vi "Synthetic_Jet_Optimisation.vi"() -> (5 "Plug in titles":string[](array[string]), 7 "Plug in values":string[](array[string]))   [LabVIEW 2011]
uses:
  Controls/SJ_Channels.ctl
  Controls/SJ_Data_Cluster.ctl
  <vilib>/Analysis/2dsp.llb/Integral Method.ctl
  Globals/Meas_global.vi
  Globals/Plug_in_data_global.vi
  <vilib>/Analysis/1siggen.llb/Ramp Pattern by Delta.vi
  <vilib>/Analysis/baseanly.llb/Scale 1D.vi
  <vilib>/Analysis/5stat.llb/RMS (DBL).vi
  <vilib>/Analysis/8numeric.llb/1D Numeric Integration.vi
  <vilib>/Analysis/baseanly.llb/Quick Scale 1D.vi
  <vilib>/Analysis/1siggen.llb/Ramp Pattern by Samples.vi
  Acquisition/Data_Translation/DataTranslation_global.vi
  <vilib>/Analysis/NI_AALBase.lvlib
  <vilib>/Analysis/NI_AALPro.lvlib
panel:
  out "subarray":dbl[][](array[numeric])
  out "output array 2":dbl[][][](array[numeric])
  out "output array":dbl[][][](array[numeric])
  out "Updated Amps":dbl[](array[numeric])
  out "Max Amp":dbl
  out "Min Amp":dbl
  out "Sweep Frequency":dbl[](array[numeric])
  out "Last Block in Genertation":bool
  out "Max Input Voltage _V_":dbl
  out "Blocks per Generation":i32
  out "Sweep Size":i32
  out "Number of Particles":i32
  out "ID Number":i32
  out "Number of Generations":i32
  out "Optimisation Type":i32
  out "Target Value":dbl
  out "Phase Average?":bool
  out "Samps per cyle":i32
  out "Formation Criteria":dbl
  out "Jet Formation":bool
  out "Strouhal Number":dbl
  out "Stokes Number":dbl
  out "nu":dbl=1.55e-05
  out "Omega":dbl=1200.0
  out "Reynolds Number":dbl
  out "Charicteristic Velocity m_s":dbl
  out "Stroke Length _m_":dbl
  out "Cavity:Helmholtz:Hz":dbl=428.16291209383184
  out "LEM Velocity _ms_":dbl[](array[numeric])=[3.7049856348371377, 3.4607988115264297, 3.0653584733968287, 2.5359472607578692, 1.895702983998723, 1.1726073902466658, 0.3982632267462864, -0.3934869508418966, -1.1680398605184126, -1.8915438234131698, -2.5323782445904723, -3.062535584780142, -3.458845424238726, -3.7039871212762807, -3.787246807411894, -3.7049856348371377, -3.4607988115264297, -3.0653584733968295, -2.5359472607578692, -1.8957029839987247, -1.172607390246666, -0.3982632267462887, 0.3934869508418962, 1.1680398605184101, 1.8915438234131694, 2.53237824459047, 3.0625355847801417, 3.4588454242387248, 3.7039871212762803, 3.7872468074118935]
  out "LEM Max Velocity _ms_":dbl=3.7872475686779676
  out "LEM Phase Velocity _deg_":dbl=-258.0363282123533
  out "Phase Pressure _deg_":dbl=-169.14507601114087
  out "Phase Velocity _deg_":dbl=373.1272896341652
  out "Phase Input Voltage _deg_":dbl=8.606071626556414
  out "Phase Angle _deg_":dbl[](array[numeric])=[0.0, 12.0, 24.0, 36.0, 48.0, 60.0, 72.0, 84.0, 96.0, 108.0, 120.0, 132.0, 144.0, 156.0, 168.0, 180.0, 192.0, 204.0, 216.0, 228.0, 240.0, 252.0, 264.0, 276.0, 288.0, 300.0, 312.0, 324.0, 336.0, 348.0]
  out "Amplitude (V)":dbl=70.0
  out "Frequency (Hz)":dbl=1200.0
  out "AS Freq":dbl=36036.04
  out "Output Data Names":string[](array[string])=["Max Pressure _Pa_", "Max Velocity m_s", "Max Current _A_", "Max Displacement _m_", "Phase Displ _deg_", "Phase Pressure _deg_", "Phase Velocity _deg_", "Phase Current _deg_", "Phase Input Voltage _deg_", "LEM Max Velocity _ms_", "LEM Phase Velocity _deg_"]
  out "Input Voltage _V_":dbl[](array[numeric])=[-5.5088632433799996, -12.651031578584, -19.235618350895997, -24.9961110527, -29.670494279084004, -33.04444558276, -35.005182361704, -35.409211536216006, -34.310616683552006, -31.700640287920002, -27.711473499856005, -22.510574222680006, -16.349366000988, -9.495663135284, -2.196569584672, 5.184714435096, 12.336113665324001, 18.917564300223997, 24.689891482827996, 29.395636083331993, 32.795741589576, 34.758786092276, 35.215182844328, 34.127830748423996, 31.539748142271996, 27.582652797175996, 22.404475723135995, 16.265220463328, 9.402109185388, 2.133489422836]
  out "Pressure _Pa_":dbl[](array[numeric])=[-27.3956675953706, 95.65286233449294, 217.28142105099454, 325.3916285730047, 412.49320713856633, 477.62511872885386, 518.8812420389512, 544.5955786383588, 546.2858417945154, 525.7943338813993, 485.98446016799124, 431.53940396868336, 357.29264741860004, 257.81676584697294, 146.44897730607346, 25.39291194062997, -95.29994862668336, -216.63005998968256, -325.4638615668826, -412.65459893301875, -477.423305725176, -519.6780076017092, -543.7330519967387, -544.6659346048561, -524.568602441649, -487.2326508157636, -435.0203186855821, -361.9795522274816, -267.2741357434412, -152.01151538796677]
  out "Zeros":dbl[](array[numeric])=[1.4978743085562871, 0.2341330189017041, -0.35175473981443495, 0.0022887999999999997, -3.0068544366899315, 2.8293]
  out "Velocity m_s":dbl[](array[numeric])=[-0.006589971422005106, -0.006419643065741468, -0.009111611844261746, -0.006030326884042168, -0.004272653157727323, -0.0068849933436421745, -0.010636233235274354, -0.0035467148583991693, -0.008496862890472292, -0.005357351691532665, -0.007065956289182962, -0.006648911559621155, -0.005058171342073957, -0.008830133605031026, -0.0038751674420970687, -0.005274584307176274, 0.000979796600094568, -0.005616008146962059, -0.00729733372181674, 0.0005036149760482819, -0.004633370846616606, -0.007598533001820504, -0.005354959759266961, -0.003855515705978843, -0.005082756078867318, -0.0008163141834672163, -0.007346968606858383, -0.00413574997102441, -0.00277648312445221, -0.00052352239052674]
  out "RMS Velocity m_s":dbl=0.014914535983039488 format="%0.2f"
  out "RMS Pressure _Pa_":dbl=395.7699897259115 format="%0.2f"
  out "Max Pressure _Pa_":dbl=546.2858417945154 format="%0.2f"
  out "Max Velocity m_s":dbl=0.000979796600094568
  in  "Menu Ring":u16(ring) items=["Max Pressure _Pa_", "", "Max Velocity m_s"]
  out "Frequency Plot":cluster{"Sweep Frequency":dbl[], dbl[]}[](graph)
  out "Pressure Plot":cluster{dbl[], dbl[]}[](graph)=[{[0.0, 12.0, 24.0, 36.0, 48.0, 60.0, 72.0, 84.0, 96.0, 108.0, 120.0, 132.0, 144.0, 156.0, 168.0, 180.0, 192.0, 204.0, 216.0, 228.0, 240.0, 252.0, 264.0, 276.0, 288.0, 300.0, 312.0, 324.0, 336.0, 348.0], [-0.15557712257291065, -0.35728080433659803, -0.5432376920119246, -0.705921142218441, -0.8379315153272326, -0.9332160799164545, -0.9885897155857659, -1.0, -0.9689743203815658, -0.8952653536353687, -0.7826063416157439, -0.6357265029653804, -0.4617263500562873, -0.2681692905127802, -0.06203384626131485, 0.1464227586596542, 0.34838713233438734, 0.5342554516040381, 0.697273122209331, 0.8301691793748806, 0.926192371045399, 0.9816311796924717, 0.9945203893712923, 0.9638122191316959, 0.8907215601232357, 0.7789682853842954, 0.632730149899583, 0.45934997583022086, 0.26552721106968635, 0.060252384345070756]}, {[0.0, 12.0, 24.0, 36.0, 48.0, 60.0, 72.0, 84.0, 96.0, 108.0, 120.0, 132.0, 144.0, 156.0, 168.0, 180.0, 192.0, 204.0, 216.0, 228.0, 240.0, 252.0, 264.0, 276.0, 288.0, 300.0, 312.0, 324.0, 336.0, 348.0], [-0.05014896140338823, 0.1750967259562854, 0.39774309423293575, 0.5956435325215701, 0.7550867615085017, 0.8743135592895557, 0.9498346878887768, 0.9969058997564276, 1.0, 0.9624894032658751, 0.8896156974736197, 0.7899516534258018, 0.6540397353973438, 0.47194480640402603, 0.2680812243366908, 0.0464828300459258, -0.17445070206035157, -0.39655074947222896, -0.5957757581594167, -0.7553821962097238, -0.87394413180629, -0.9512932019153176, -0.9953270072140422, -0.9970346894139926, -0.9602456485390019, -0.8919005647578826, -0.7963236192550169, -0.6626193185574809, -0.4892569334498257, -0.2782636922981901]}]
  out "Velocity Plot":cluster{dbl[], dbl[]}[](graph)=[{[0.0, 12.0, 24.0, 36.0, 48.0, 60.0, 72.0, 84.0, 96.0, 108.0, 120.0, 132.0, 144.0, 156.0, 168.0, 180.0, 192.0, 204.0, 216.0, 228.0, 240.0, 252.0, 264.0, 276.0, 288.0, 300.0, 312.0, 324.0, 336.0, 348.0], [-0.15557712257291065, -0.35728080433659803, -0.5432376920119246, -0.705921142218441, -0.8379315153272326, -0.9332160799164545, -0.9885897155857659, -1.0, -0.9689743203815658, -0.8952653536353687, -0.7826063416157439, -0.6357265029653804, -0.4617263500562873, -0.2681692905127802, -0.06203384626131485, 0.1464227586596542, 0.34838713233438734, 0.5342554516040381, 0.697273122209331, 0.8301691793748806, 0.926192371045399, 0.9816311796924717, 0.9945203893712923, 0.9638122191316959, 0.8907215601232357, 0.7789682853842954, 0.632730149899583, 0.45934997583022086, 0.26552721106968635, 0.060252384345070756]}, {[0.0, 12.0, 24.0, 36.0, 48.0, 60.0, 72.0, 84.0, 96.0, 108.0, 120.0, 132.0, 144.0, 156.0, 168.0, 180.0, 192.0, 204.0, 216.0, 228.0, 240.0, 252.0, 264.0, 276.0, 288.0, 300.0, 312.0, 324.0, 336.0, 348.0], [-0.0017400427690923374, -0.0016950685794170583, -0.002405866928563968, -0.0015922719565676093, -0.001128168660507009, -0.0018179415532591603, -0.002808434141249664, -0.0009364889690996669, -0.002243546122698781, -0.0014145768585897204, -0.0018657237429983216, -0.001755605561963586, -0.0013355800662831847, -0.0023315442732039188, -0.0010232149208002786, -0.001392722622896813, 0.00025870946624789303, -0.0014828735576385352, -0.0019268175782828233, 0.00013297653986074366, -0.0012234140213805954, -0.002006347457194939, -0.0014139452830977239, -0.0010180259967302217, -0.001342071519849202, -0.00021554290622666447, -0.0019399233745421283, -0.001092020188103525, -0.0007331138596561618, -0.00013823297428152076]}, {[0.0, 12.0, 24.0, 36.0, 48.0, 60.0, 72.0, 84.0, 96.0, 108.0, 120.0, 132.0, 144.0, 156.0, 168.0, 180.0, 192.0, 204.0, 216.0, 228.0, 240.0, 252.0, 264.0, 276.0, 288.0, 300.0, 312.0, 324.0, 336.0, 348.0], [0.9782794265180274, 0.9138033477917035, 0.8093896778519208, 0.6696017951074252, 0.5005491008108334, 0.3096200089077361, 0.10515903689372944, -0.10389788964157722, -0.3084139798421589, -0.49945089918916635, -0.6686594176102914, -0.8086443108979737, -0.9132875674934984, -0.9780157749495838, -1.0, -0.9782794265180274, -0.9138033477917035, -0.8093896778519211, -0.6696017951074252, -0.5005491008108338, -0.30962000890773617, -0.10515903689373006, 0.10389788964157712, 0.3084139798421583, 0.4994508991891662, 0.6686594176102908, 0.8086443108979736, 0.9132875674934979, 0.9780157749495837, 0.9999999999999999]}]
  out "Amplitude String":string="3.5000"
  out "Frequency String":string="1200"
  # "You Must have selected the \"Save Data\" option on the \nMeasurement Program for this vi to work correctly"
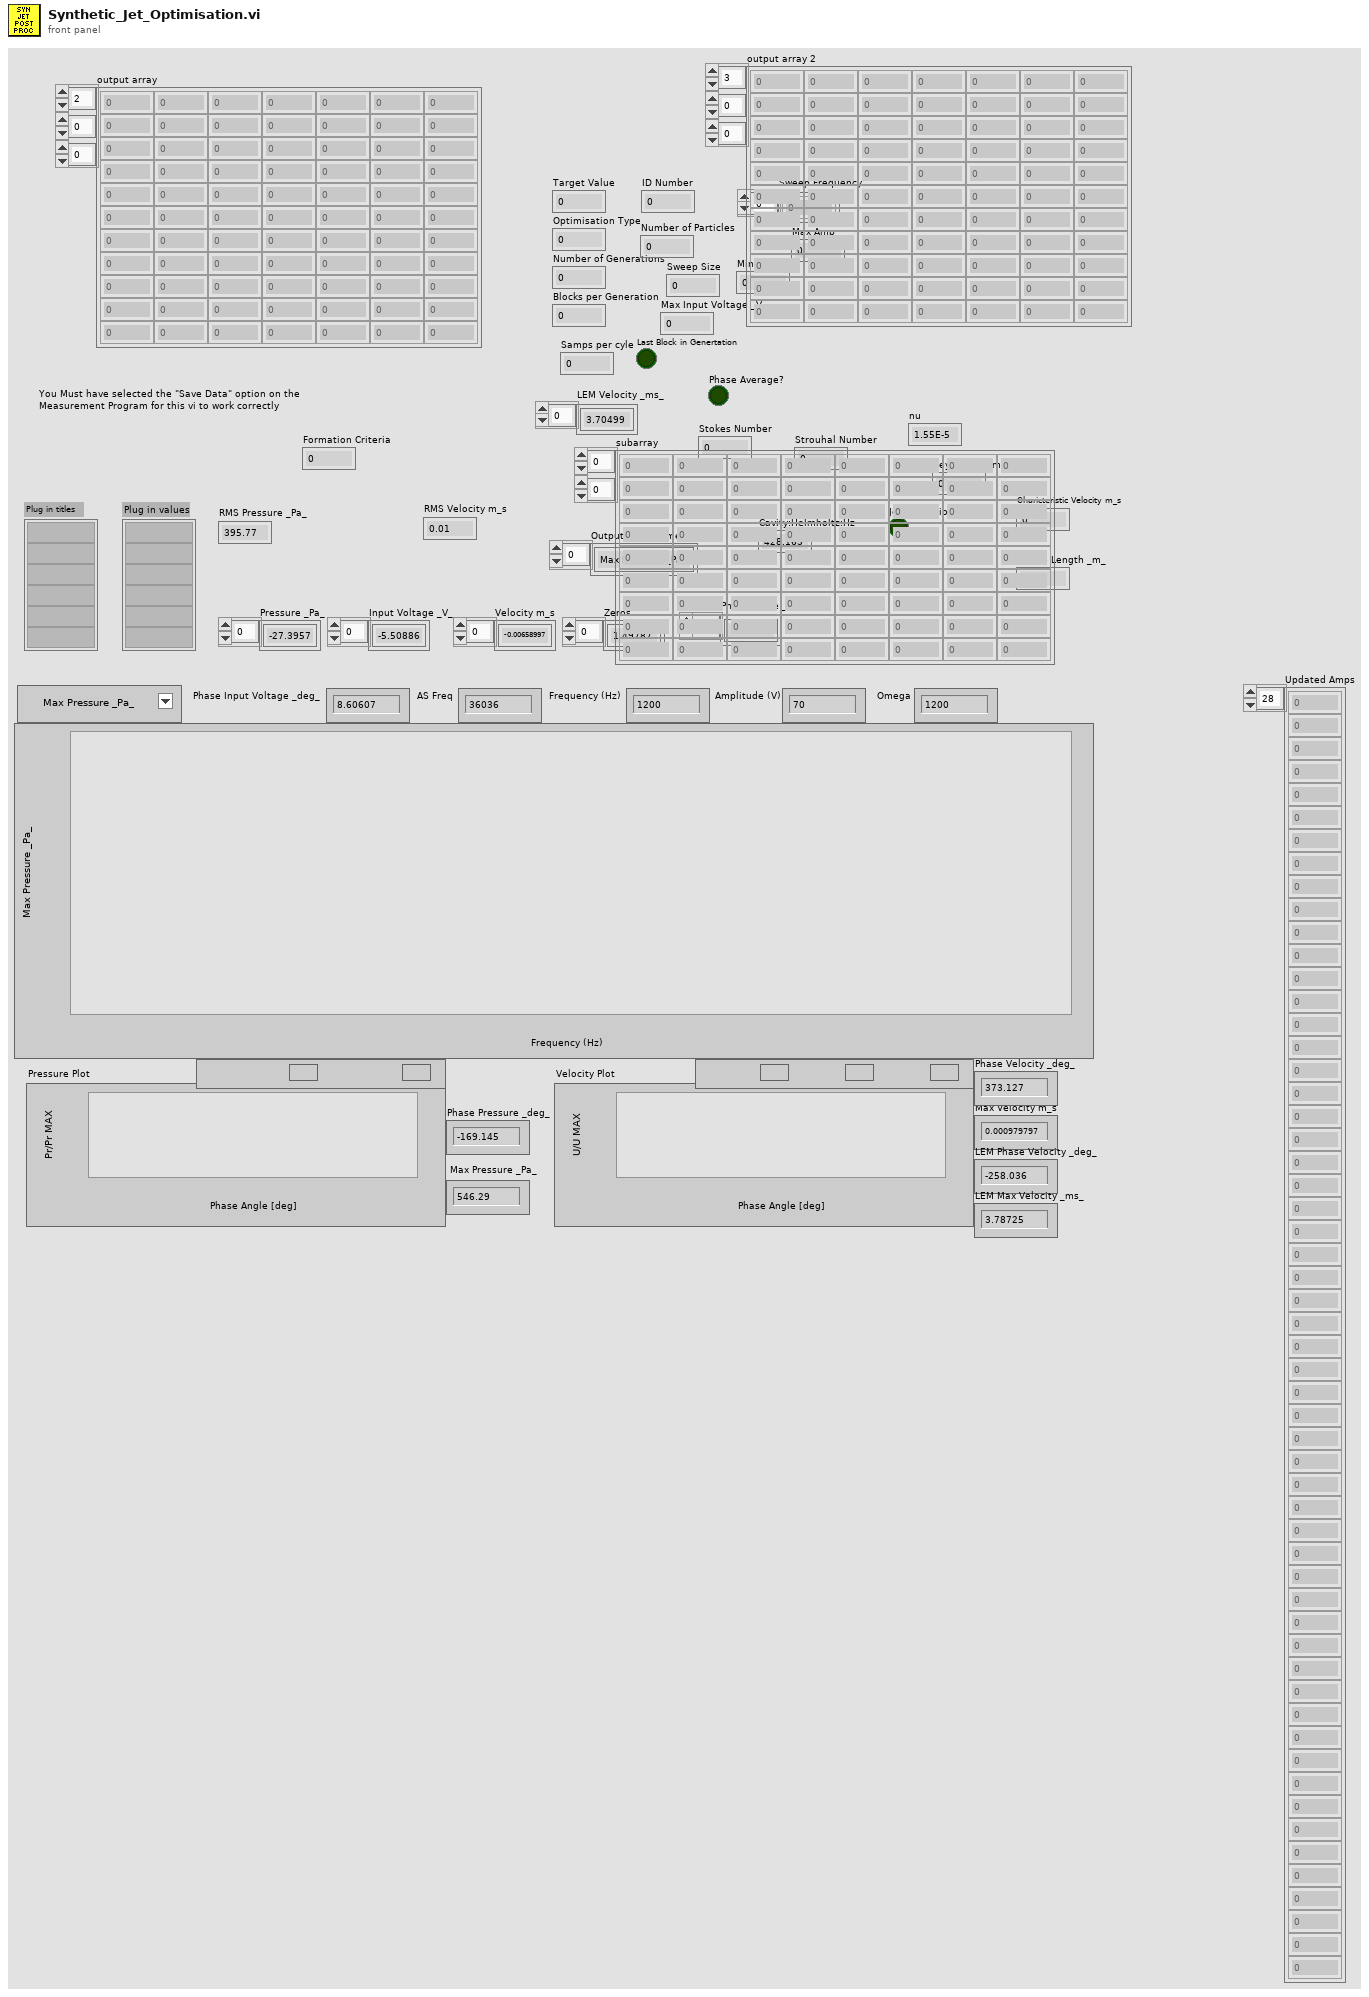
[diagram p1: front panel]
types:
  T1 = typedef "SJ_Channels.ctl" = string[]
  T2 = typedef "Analysis_info_cluster.ctl" = cluster{"Colour":u32, "Inst type":T3, "Inst name":string, "Symbol":string, "Code name":string, "Extra Info":string, "Inst Array":T4, "Index":i32, "Voltage Index":i32, "Extra Titles":string[], "Extra Values":string[]}
  T3 = typedef "Inst_type.ctl" = enum16{"Propeller anemometer", "Raw voltage", "Pressure Transducer", "Pitot-static tube", "Preston tube", "Hot wire", "Cross wire 1", "Cross wire 2", "Generic Linear", "Generic Polynomial", "Generic BackPoly", "Fast FID", "Thermocouple", "Cold wire", "Pulsed Wire", "LDA Vel", "LDA Tran time", "LDA Arr time"}
  T4 = typedef "Instrument_Array.ctl" = enum16{"PWA", "LDA", "Analogue"}
  T5 = typedef "Post_Process.ctl" = enum16{"Take New Data", "Post Process Raw Data File"}
  T6 = cluster{"Name":string, "X":dbl, "Y":dbl, "Z":dbl}[]
  T7 = typedef "SJ_Data_Cluster.ctl" = cluster{"Do":dbl, "Dc":dbl, "Ho":dbl, "Hc":dbl, "K":dbl, "beta":dbl, "Vc":dbl, "Vo":dbl}
  T8 = cluster{"R":dbl, "Mair":dbl, "T":dbl, "Patmos":dbl, "gamma":dbl}
  T9 = typedef "NI_AALPro.lvlib/Integral Method.ctl" = i32
  T10 = cluster{"Ramp Pattern":dbl[], "Y[i]=X[i]/Max|X|":dbl[]}
  T11 = cluster{"Ramp Pattern":dbl[], "Y[i]=X[i]/Max|X|":dbl[]}[]
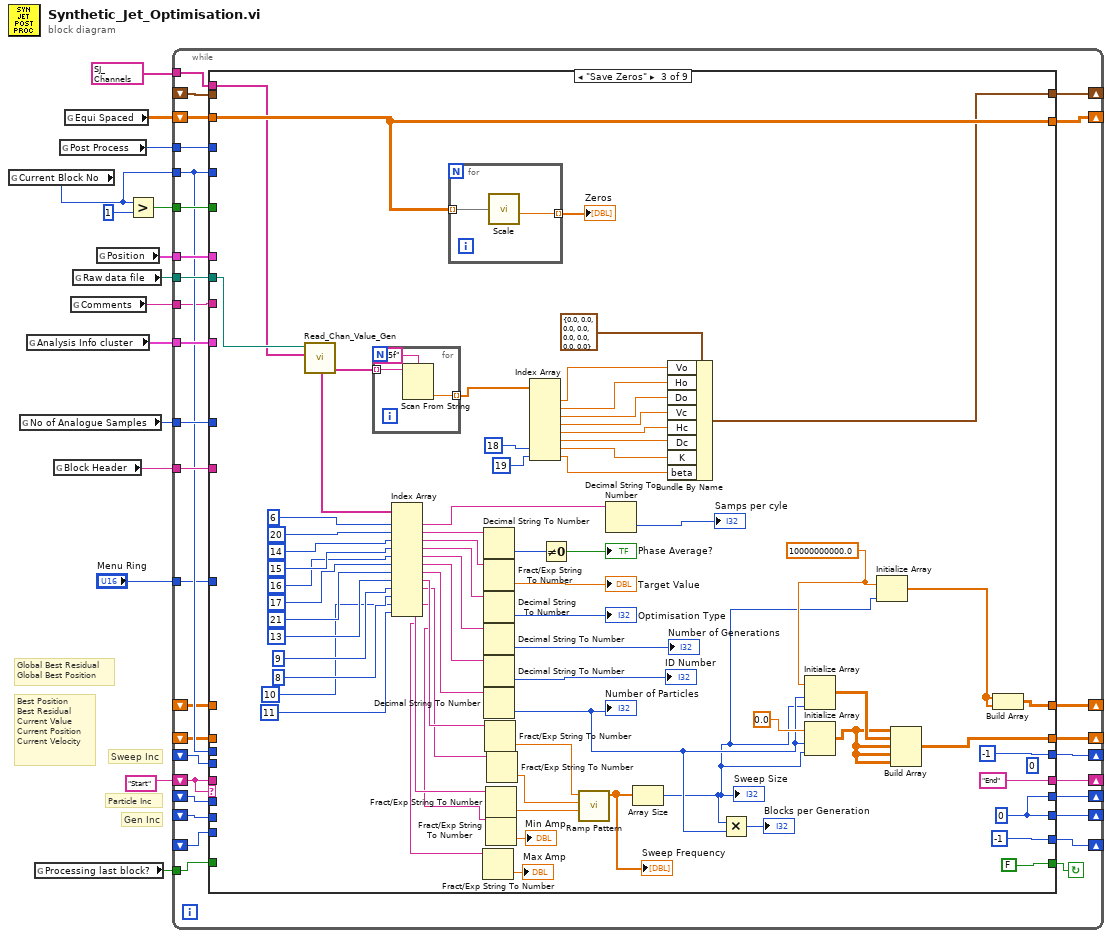
[diagram p0: block diagram]
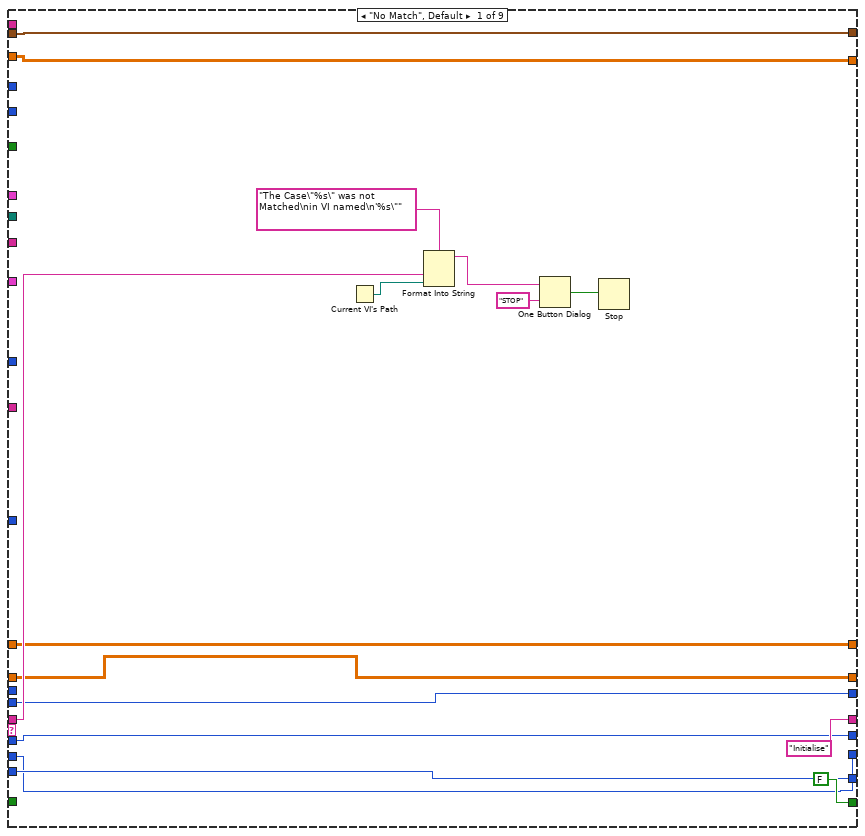
[diagram p2: hidden frame]
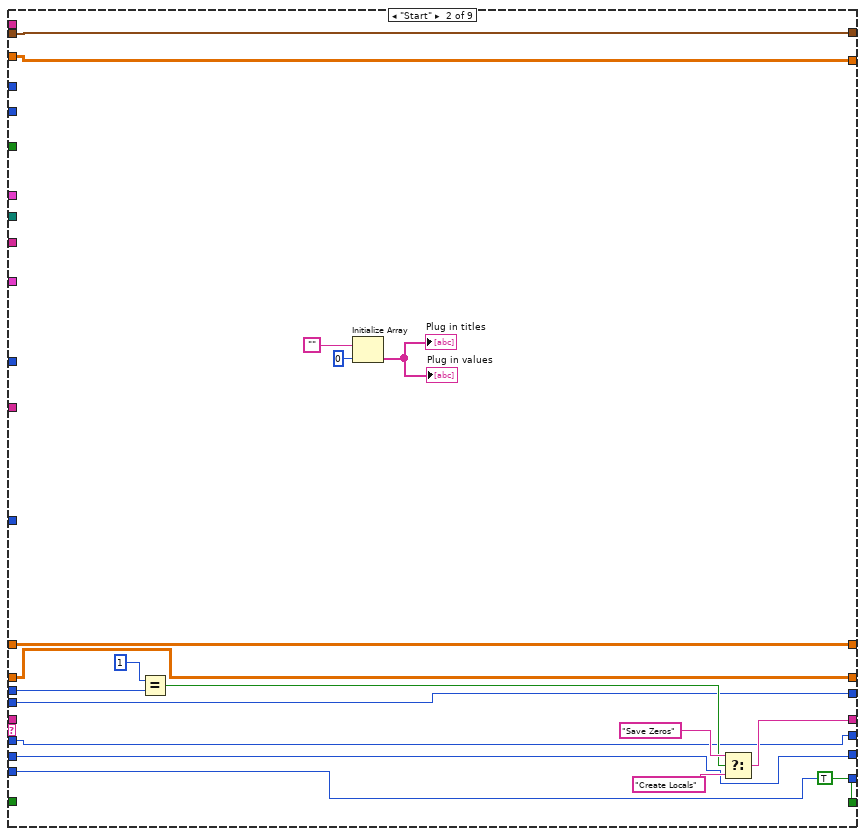
[diagram p3: hidden frame]
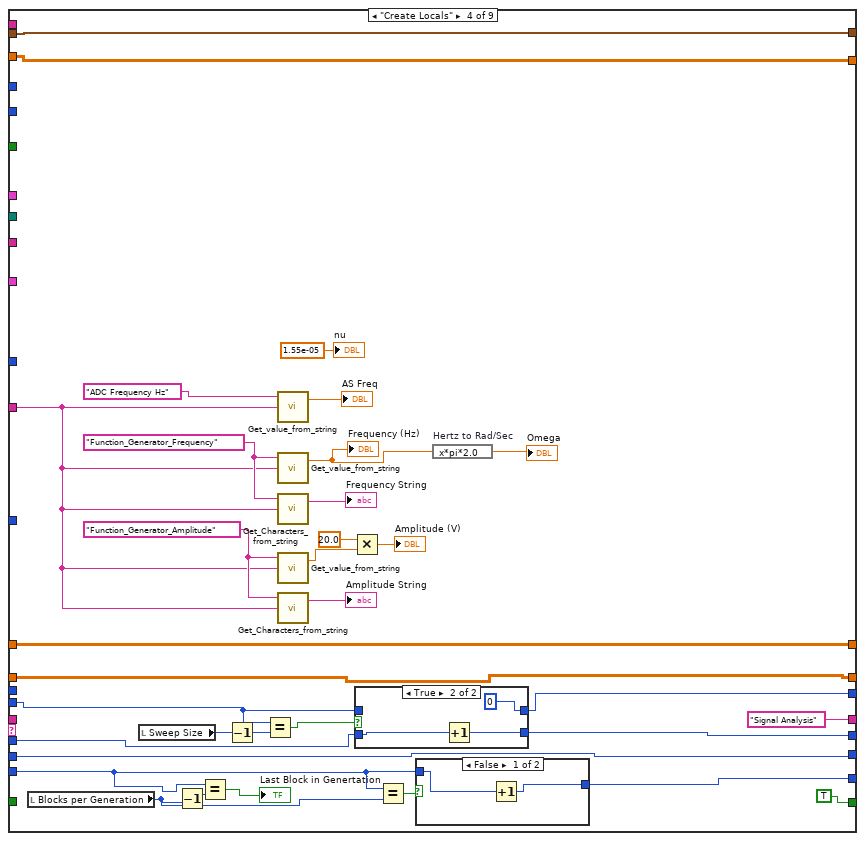
[diagram p4: hidden frame]
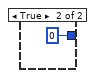
[diagram p5: hidden frame]
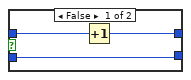
[diagram p6: hidden frame]
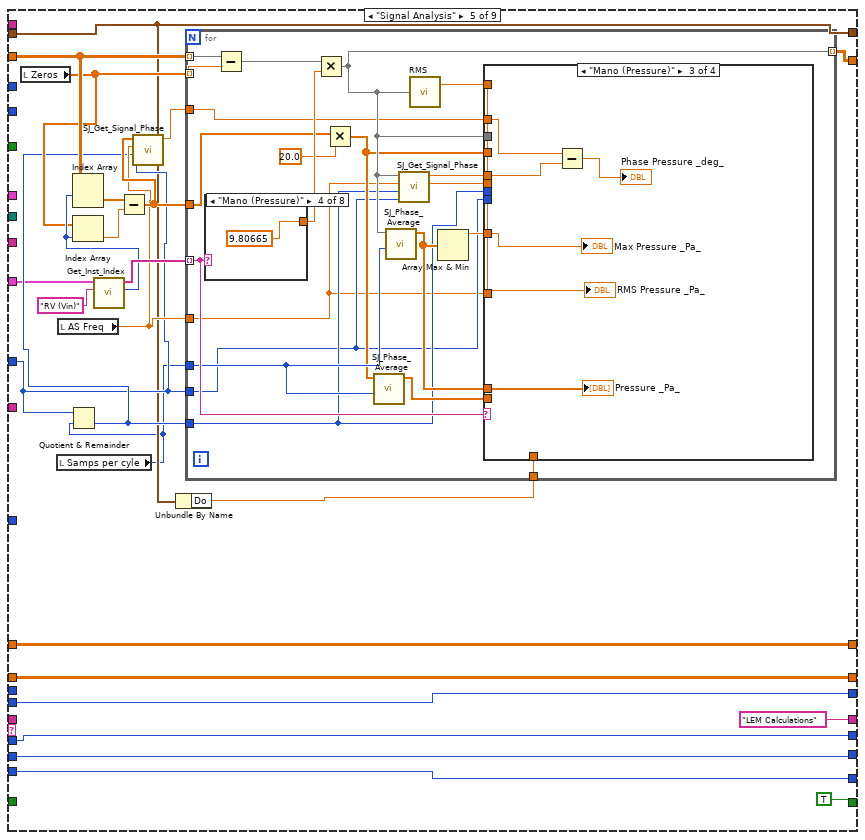
[diagram p7: hidden frame]
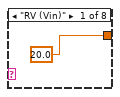
[diagram p8: hidden frame]
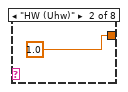
[diagram p9: hidden frame]
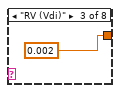
[diagram p10: hidden frame]
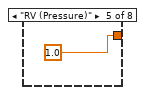
[diagram p11: hidden frame]
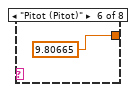
[diagram p12: hidden frame]
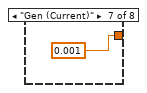
[diagram p13: hidden frame]
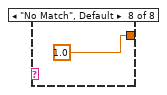
[diagram p14: hidden frame]
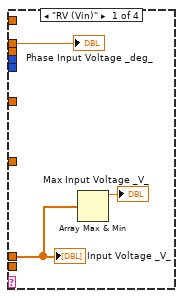
[diagram p15: hidden frame]
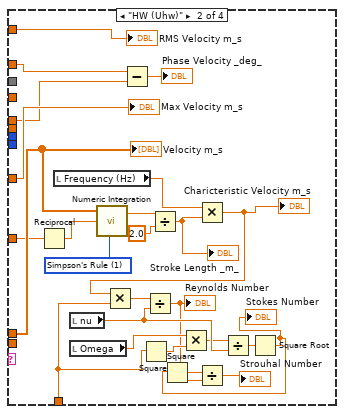
[diagram p16: hidden frame]
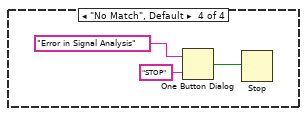
[diagram p17: hidden frame]
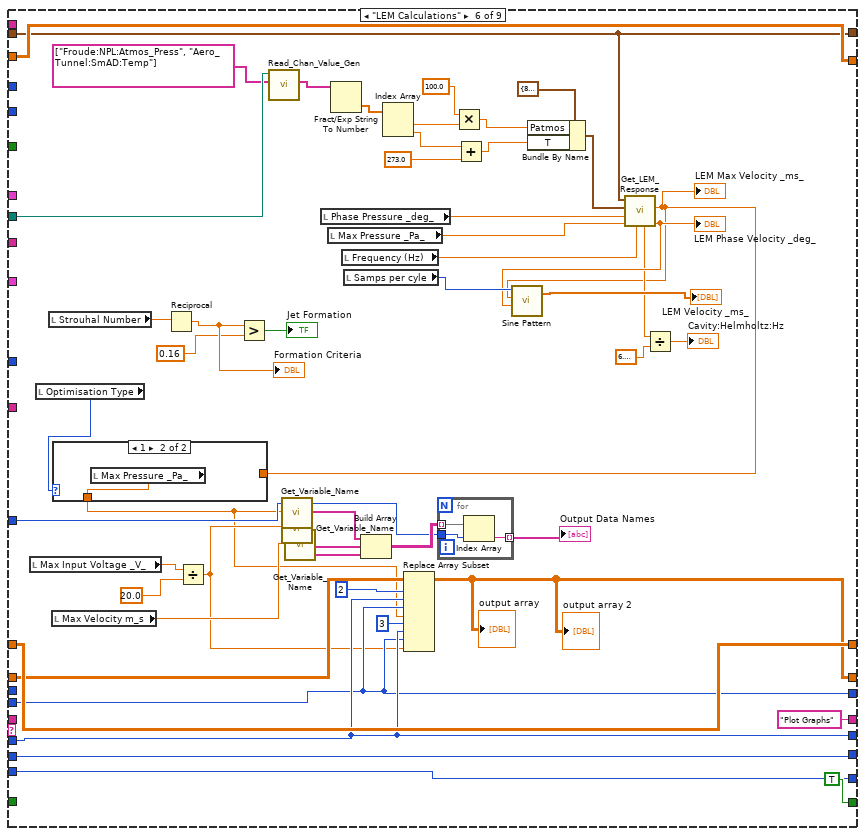
[diagram p18: hidden frame]
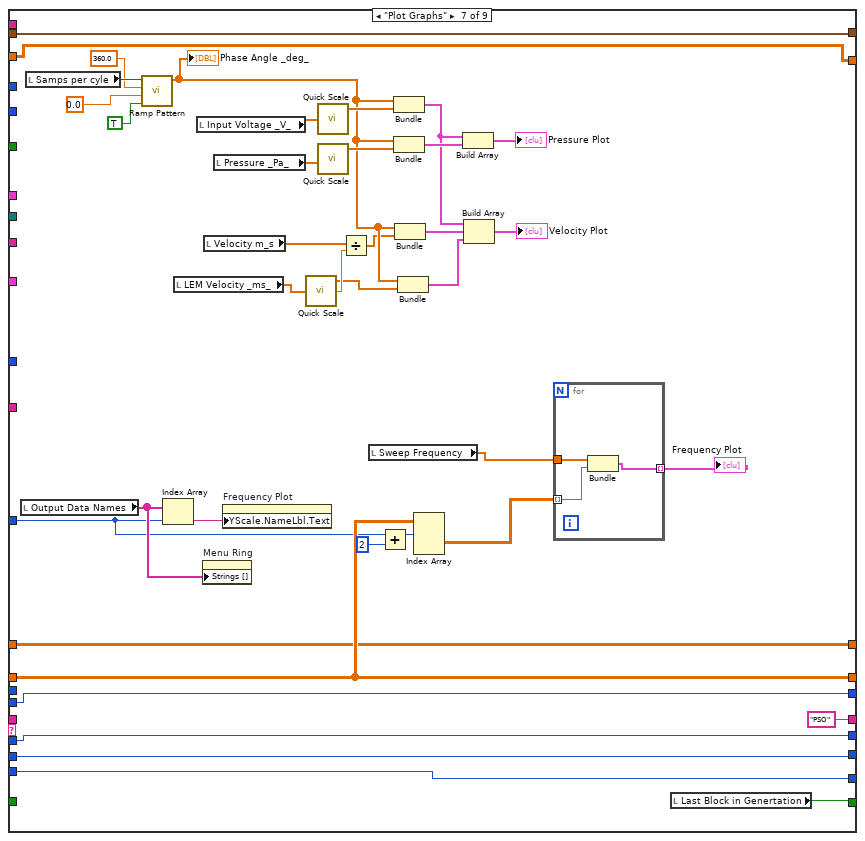
[diagram p20: hidden frame]
diagram:
  # "Particle Inc"
  # "Gen Inc"
  # "Sweep Inc"
  # "Global Best Residual\nGlobal Best Position"
  # "Best Position\nBest Residual\nCurrent Value\nCurrent Position\nCurrent Velocity"
  n1 = global read "Meas_global.vi" "Current Block No"() -> (w11:i32)
  n2 = global read "Meas_global.vi" "No of Analogue Samples"() -> (w7:i32)
  n3 = global read "Meas_global.vi" "Analysis Info cluster"() -> (w10:T2[])
  n4 = global read "Meas_global.vi" "Processing last block?"() -> (w5:bool)
  n5 = global read "Plug_in_data_global.vi" "Block Header"() -> (w8:string)
  n6 = global read "Meas_global.vi" "Post Process"() -> (w2:T5)
  n7 = global read "Plug_in_data_global.vi" "Equi Spaced"() -> (w9:dbl[][])
  n8 = global read "Meas_global.vi" "Comments"() -> (w4:string)
  n9 = global read "Meas_global.vi" "Raw data file"() -> (w14:path)
  n10 = global read "Meas_global.vi" "Position"() -> (w6:T6)
  n11 = Greater?(x=w11, y=1) -> (0:w12:bool)
  n12 = while {
    shift-left: "Start" -> [w46]
    shift-right: [w36] -> _
    tunnel: w14 -> [w45]
    tunnel: w12 -> [w44]
    tunnel: w11 -> [w37]
    tunnel: w10 -> [w43]
    tunnel: w8 -> [w41]
    tunnel: w7 -> [w40]
    tunnel: w6 -> [w39]
    tunnel: w5 -> [w38]
    shift-right: [w34] -> _
    shift-left: w9 -> [w42]
    tunnel: w4 -> [w33]
    tunnel: "Menu Ring" -> [w32]
    tunnel: w2 -> [w31]
    shift-right: [w29] -> _
    shift-left: _ -> [w30]
    tunnel: T1 ["Synthetic_Jet:Orifice:Volume", "Synthetic_Jet:Orifice:Height", "Synthetic_Jet:Orifice:Diameter", "Synthetic_Jet:Cavity:Volume", "Synthetic_Jet:Cavity:Height", "Synthetic_Jet:Cavity:Diameter", "Synthetic_Jet:Samples:Per_Cycle", "Synthetic_Jet:Dwell:Time", "Synthetic_Jet:Minimum:Frequency", "Synthetic_Jet:Maximum:Frequency", "Synthetic_Jet:Minimum:Amplitude", "Synthetic_Jet:Maximum:Amplitude", "Synthetic_Jet:Amplitude:Delta", "Synthetic_Jet:Frequency:Delta", "Synthetic_Jet:Calibration:Velocity", "Synthetic_Jet:Calibration:Type", "Synthetic_Jet:Calibration:No_Of_Gens", "Synthetic_Jet:Identification:Number", "Synthetic_Jet:LEM_Pressure:Coefficient", "Synthetic_Jet:LEM_Added_Mass:Coefficient", "Synthetic_Jet:Phase:Average?", "Synthetic_Jet:Optimisation:Particles"] ("Synthetic Jet Specific Channels") -> [w28]
    shift-right: [w27] -> _
    shift-left: _ -> [w26]
    shift-right: [w25] -> _
    shift-left: _ -> [w24]
    shift-right: [w23] -> _
    shift-left: _ -> [w22]
    shift-right: [w21] -> _
    shift-left: _ -> [w20]
    shift-right: [w19] -> _
    shift-left: _ -> [w18]
    shift-right: [w17] -> _
    shift-left: _ -> [w16]
    stop <- w35 continue-if-true
    n13 = case shown="\"Save Zeros\"" w46 {
      tunnel: w46 -> [w58 _ _ _ _ _ _ _ _]
      tunnel: w45 -> [_ _ w144 _ _ w316 _ _ _]
      tunnel: w44 -> [_ _ _ _ _ _ _ _ _]
      tunnel: w37 -> [_ _ _ _ _ _ _ _ _]
      tunnel: w43 -> [_ _ _ _ w207 _ _ _ _]
      tunnel: w42 -> [w54 w71 w147 w180 w214 w335 w371 w433 w467]
      tunnel: w41 -> [_ _ _ w183 _ _ _ _ _]
      tunnel: w40 -> [_ _ _ _ w209 _ _ _ _]
      tunnel: w39 -> [_ _ _ _ _ _ _ _ _]
      tunnel: w38 -> [_ _ _ _ _ _ _ w432 _]
      tunnel: w37 -> [_ w77 _ _ _ _ _ _ _]
      tunnel: ["Initialise" w73 "End" ("t") "Signal Analysis" "LEM Calculations" "Plot Graphs" "PSO" "End" ("t") "" ("t")] -> w36
      tunnel: [FALSE TRUE FALSE TRUE TRUE TRUE ("Processing last block?") w351 w432 FALSE ("Processing last block?")] -> w35
      tunnel: [w54 w71 w147 w180 w220 w335 w371 w433 w467] -> w34
      tunnel: w33 -> [_ _ _ _ _ _ _ _ _]
      tunnel: w32 -> [_ _ _ _ _ w297 w353 _ _]
      tunnel: w31 -> [_ _ _ _ _ _ _ _ _]
      tunnel: w30 -> [w53 w69 _ w172 w206 w320 w364 w437 w468]
      tunnel: [w53 w69 w145 w172 w206 w320 w364 w437 w468] -> w29
      tunnel: w28 -> [_ _ w143 _ _ _ _ _ _]
      tunnel: [w52 w67 w95 w159 w203 w293 w354 w430 w466] -> w27
      tunnel: w26 -> [w52 w67 _ w159 w203 w296 w354 w431 w466]
      tunnel: [w51 w68 -1 ("index") w171 w202 w291 w357 w434 w465] -> w25
      tunnel: w24 -> [w51 w68 _ w170 w202 w291 w357 w434 w465]
      tunnel: [w50 w66 -1 ("index") w167 w201 w309 w356 w436 w464] -> w23
      tunnel: w22 -> [w50 w66 _ w156 w201 w309 w356 w436 w464]
      tunnel: [w49 w65 w92 w163 w200 w301 w352 w415 w461] -> w21
      tunnel: w20 -> [w49 w65 _ w163 w200 w301 w352 w422 w461]
      tunnel: [w48 w64 w84 w162 w199 w299 w350 w391 w460] -> w19
      tunnel: w18 -> [w48 w64 _ w162 w199 w299 w350 w389 w460]
      tunnel: [w47 w63 w84 w161 w198 w292 w348 0 ("index") w459] -> w17
      tunnel: w16 -> [w47 w63 _ w160 w198 w292 w348 _ w459]
      frame "No Match", Default {
        n14 = Current VI's Path() -> (path=w57:path)
        n15 = Format Into String(format string="The Case\"%s\" was not Matched\nin VI named\n'%s\"" ("Format String"), w58, w57) -> (resulting string=w61:string)  [unwired: 2 in, 1 out]
        n16 = One Button Dialog(message=w61, button name ("OK")="STOP") -> (true=w59:bool)
        n17 = Stop(stop? (T)=w59) -> ()
      }
      frame "Start" {
        n18 = Equal?(x=1, y=w77) -> (x = y?=w70:bool)
        n19 = Initialize Array("", 0) -> (→"Plug in values" →"Plug in titles":string[])
        n20 = Select(t="Save Zeros", s=w70, f="Create Locals") -> (s? t:f=w73:string)
      }
      frame "Save Zeros" {
        w84 = 0 ("index")
        w94 = 10000000000.0
        (unwired) 0 ("index")
        (unwired) FALSE ("Processing last block?")
        (unwired) "End" ("t")
        (unwired) "End" ("t")
        (unwired) FALSE ("Processing last block?")
        n21 = call "Read_Chan_Value_Gen.vi"("Desired Ch Names"=w143, "Raw data file"=w144) -> ("Values"=w123:string[])  [unwired: 9 in]
        n22 = for {
          tunnel: w123 -> [w153] mode=indexing
          tunnel: [w151] -> w132 mode=indexing
          n23 = Scan From String(format string="%5f", input string=w153) -> (output 1=w151:dbl)  [unwired: 3 in, 3 out]
        }
        n24 = Index Array(array=w123, index #1=6 ("index"), index #2=20 ("index"), index #3=14 ("index"), index #4=15 ("index"), index #5=16 ("index"), index #6=17 ("index"), index #7=21 ("index"), index #8=13 ("index"), index #9=9 ("index"), index #10=8 ("index"), index #11=10 ("index"), index #12=11 ("index")) -> (element #1=w130:string, element #2=w121:string, element #3=w120:string, element #4=w119:string, element #5=w118:string, element #6=w117:string, element #7=w116:string, element #8=w106:string, element #9=w105:string, element #10=w104:string, element #11=w88:string, element #12=w87:string)
        n25 = for {
          tunnel: w147 -> [w155] mode=indexing
          tunnel: [w154] -> w149 mode=indexing
          n26 = call-poly <vilib>:"Scale.vi"("X"=w155) -> ("offset"=w154:dbl)  [unwired: 3 out]
        }
        "Zeros" <- w149
        n27 = Fract/Exp String To Number(string=w87) -> (number=→"Max Amp":dbl)  [unwired: 3 in, 1 out]
        n28 = Decimal String To Number(string=w121) -> (number=w128:i32)  [unwired: 2 in, 1 out]
        n29 = Fract/Exp String To Number(string=w120) -> (number=→"Target Value":dbl)  [unwired: 3 in, 1 out]
        n30 = Decimal String To Number(string=w119) -> (number=→"Optimisation Type":i32)  [unwired: 2 in, 1 out]
        n31 = Decimal String To Number(string=w118) -> (number=→"Number of Generations":i32)  [unwired: 2 in, 1 out]
        n32 = Decimal String To Number(string=w117) -> (number=→"ID Number":i32)  [unwired: 2 in, 1 out]
        n33 = Decimal String To Number(string=w116) -> (number=w82:i32)  [unwired: 2 in, 1 out]
        "Number of Particles" <- w82
        n34 = Fract/Exp String To Number(string=w106) -> (number=w103:dbl)  [unwired: 3 in, 1 out]
        n35 = Fract/Exp String To Number(string=w104) -> (number=w101:dbl)  [unwired: 3 in, 1 out]
        n36 = Fract/Exp String To Number(string=w88) -> (number=→"Min Amp":dbl)  [unwired: 3 in, 1 out]
        n37 = Fract/Exp String To Number(string=w105) -> (number=w102:dbl)  [unwired: 3 in, 1 out]
        n38 = Index Array(array=w132, index #7=18 ("index"), index #8=19 ("index")) -> (element #1=w142:dbl, element #2=w141:dbl, element #3=w140:dbl, element #4=w139:dbl, element #5=w138:dbl, element #6=w137:dbl, element #7=w134:dbl, element #8=w133:dbl)  [unwired: 6 in]
        n39 = Not Equal To 0?(x=w128) -> (x != 0?=→"Phase Average?":bool)
        n40 = call-poly <vilib>:"Ramp Pattern.vi"("start"=w101, "end"=w102, "delta"=w103) -> ("Ramp Pattern"=w100:dbl[])  [unwired: 6 in, 2 out]
        "Sweep Frequency" <- w100
        n41 = Decimal String To Number(string=w130) -> (number=→"Samps per cyle":i32)  [unwired: 2 in, 1 out]
        n42 = Array Size(array=w100) -> (size(s)=w81:i32)
        "Sweep Size" <- w81
        n43 = Bundle By Name(cluster=T7 {"Do"=0.0, "Dc"=0.0, "Ho"=0.0, "Hc"=0.0, "K"=0.0, "beta"=0.0, "Vc"=0.0, "Vo"=0.0} ("SJ_Data_Cluster"), "Vo"=w142, "Ho"=w141, "Do"=w140, "Vc"=w139, "Hc"=w138, "Dc"=w137, "K"=w134, "beta"=w133) -> (w145:T7)
        n44 = Multiply(x=w81, y=w82) -> (x*y=→"Blocks per Generation":i32)
        n45 = Initialize Array(w94, w82, w81) -> (w91:dbl[][])
        n46 = Initialize Array(0.0 ("element"), w82, w81) -> (w83:dbl[][])
        n47 = Initialize Array(w94, w81) -> (w93:dbl[])
        n48 = Build Array(w83, w91, w83, w83, w83) -> (w95:dbl[][][])
        n49 = Build Array(w93, w93) -> (w92:dbl[][])
      }
      frame "Create Locals" {
        w185 = "Function_Generator_Amplitude" ("Variable name")
        w186 = "Function_Generator_Frequency" ("Variable name")
        n50 = local read "Blocks per Generation"() -> (w165:i32)
        n51 = local read "Sweep Size"() -> (w169:i32)
        n52 = Decrement(x=w165) -> (x-1=w157:i32)
        n53 = Equal?(x=w156, y=w157) -> (x = y?=→"Last Block in Genertation":bool)
        n54 = Decrement(x=w169) -> (x-1=w158:i32)
        n55 = Equal?(x=w170, y=w158) -> (x = y?=w168:bool)
        n56 = call "Get_value_from_string.vi"("Input string"=w183, "Variable name"="ADC Frequency Hz") -> ("Value"=→"AS Freq":dbl)  [unwired: 1 in, 1 out]
        n57 = call "Get_value_from_string.vi"("Input string"=w183, "Variable name"=w186) -> ("Value"=w175:dbl)  [unwired: 1 in, 1 out]
        "Frequency (Hz)" <- w175
        n58 = call "Get_Characters_from_string.vi"("Input string"=w183, "Variable name"=w186) -> ("Value"=→"Frequency String":string)  [unwired: 1 in, 1 out]
        n59 = call "Get_value_from_string.vi"("Input string"=w183, "Variable name"=w185) -> ("Value"=w178:dbl)  [unwired: 1 in, 1 out]
        n60 = call "Get_Characters_from_string.vi"("Input string"=w183, "Variable name"=w185) -> ("Value"=→"Amplitude String":string)  [unwired: 1 in, 1 out]
        n61 = Multiply(x=20.0, y=w178) -> (x*y=→"Amplitude (V)":dbl)
        n62 = case shown="True" w168 {
          tunnel: [w193 0 ("index")] -> w171
          tunnel: w170 -> [w194 _]
          tunnel: [w192 w195] -> w161
          tunnel: w160 -> [w192 w196]
          frame False {
            n63 = Increment(x=w194) -> (x+1=w193:i32)
          }
          frame True {
            n64 = Increment(x=w196) -> (x+1=w195:i32)
          }
        }
        n65 = Equal?(x=w156, y=w165) -> (x = y?=w166:bool)
        n66 = case shown="False" w166 {
          tunnel: [w189 0 ("index")] -> w167
          tunnel: w156 -> [w190 _]
          frame False {
            n67 = Increment(x=w190) -> (x+1=w189:i32)
          }
          frame True {
          }
        }
        n68 = expression code="x*pi*2.0" "Hertz to Rad/Sec"(w175) -> (→"Omega":dbl)
        "nu" <- 1.55e-05 ("y")
      }
      frame "Signal Analysis" {
        n69 = local read "Zeros"() -> (w213:dbl[])
        n70 = local read "Samps per cyle"() -> (w204:i32)
        n71 = local read "AS Freq"() -> (w211:dbl)
        n72 = Quotient & Remainder(x=w209, y=w204) -> (floor(x/y)=w210:i32)  [unwired: 1 out]
        n73 = call "Get_Inst_Index.vi"("Inst name search"="RV (Vin)" ("element"), "Analysis Info cluster"=w207) -> ("Index of Instance"=w215:i32, "Inst Name Array"=w218:string[])  [unwired: 7 in, 1 out]
        n74 = Index Array(array=w214, index (row)=w215) -> (element=w216:dbl[])  [unwired: 1 in]
        n75 = Index Array(array=w213, index=w215) -> (element=w217:dbl)
        n76 = Subtract(x=w216, y=w217) -> (x-y=w212:dbl[])
        n77 = call "SJ_Get_Signal_Phase.vi"("No of Analogue Samples"=w209, "Number of Cycles"=w210, "Actual Sampling Frequency"=w211, "Signal"=w212) -> ("Phase Angle _deg_"=w208:dbl)  [unwired: 7 in]
        n78 = Unbundle By Name(w206) -> ("Do"=w205:dbl)
        n79 = for {
          tunnel: w214 -> [w242] mode=indexing
          tunnel: w213 -> [w241] mode=indexing
          tunnel: [w230] -> w220 mode=indexing
          tunnel: w218 -> [w239] mode=indexing
          tunnel: w204 -> [w232]
          tunnel: w211 -> [w224]
          tunnel: w209 -> [w227]
          tunnel: w210 -> [w228]
          tunnel: w212 -> [w226]
          tunnel: w208 -> [w225]
          tunnel: w205 -> [w223]
          n80 = case shown="\"Mano (Pressure)\"" w239 {
            tunnel: [20.0 1.0 0.002 9.80665 1.0 9.80665 0.001 1.0] -> w237
            frame "RV (Vin)" {
            }
            frame "HW (Uhw)" {
            }
            frame "RV (Vdi)" {
            }
            frame "Mano (Pressure)" {
            }
            frame "RV (Pressure)" {
            }
            frame "Pitot (Pitot)" {
            }
            frame "Gen (Current)" {
            }
            frame "No Match", Default {
            }
          }
          n81 = Subtract(x=w242, y=w241) -> (x-y=w240:dbl[])
          n82 = Multiply(x=w240, y=w237) -> (x*y=w230:dbl[])
          n83 = Multiply(x=w226, y=20.0) -> (x*y=w229:dbl[])
          n84 = call "SJ_Phase_Average.vi"("No. of Bins"=w232, "1D Signal"=w229) -> ("Phase Averaged Signal"=w235:dbl[])  [unwired: 7 in, 2 out]
          n85 = call "SJ_Phase_Average.vi"("No. of Bins"=w232, "1D Signal"=w230) -> ("Phase Averaged Signal"=w234:dbl[])  [unwired: 7 in, 2 out]
          n86 = call "SJ_Get_Signal_Phase.vi"("No of Analogue Samples"=w227, "Number of Cycles"=w228, "Actual Sampling Frequency"=w224, "Signal"=w230) -> ("Phase Angle _deg_"=w231:dbl)  [unwired: 7 in]
          n87 = call-poly <vilib>:"RMS.vi"("X"=w230) -> ("rms value"=w238:dbl)  [unwired: 1 out]
          n88 = Array Max & Min(array=w234) -> (max value=w233:dbl)  [unwired: 3 out]
          n89 = case shown="\"Mano (Pressure)\"" w239 {
            tunnel: w234 -> [w252 w273 w284 _]
            tunnel: w235 -> [_ _ _ _]
            tunnel: w238 -> [_ w278 w283 _]
            tunnel: w233 -> [_ w277 w282 _]
            tunnel: w231 -> [w253 w276 w280 _]
            tunnel: w230 -> [_ _ _ _]
            tunnel: w229 -> [_ _ _ _]
            tunnel: w224 -> [_ _ _ _]
            tunnel: w228 -> [_ _ _ _]
            tunnel: w227 -> [_ _ _ _]
            tunnel: w225 -> [_ w275 w281 _]
            tunnel: w224 -> [_ w271 _ _]
            tunnel: w223 -> [_ w262 _ _]
            frame "RV (Vin)" {
              n90 = Array Max & Min(array=w252) -> (max value=→"Max Input Voltage _V_":dbl)  [unwired: 3 out]
              "Input Voltage _V_" <- w252
              "Phase Input Voltage _deg_" <- w253
            }
            frame "HW (Uhw)" {
              w272 = T9 1 items=["Trapezoidal Rule", "Simpson's Rule", "Simpson's 3/8 Rule", "Bode Rule"] ("integration method")
              n91 = Reciprocal(x=w271) -> (1/x=w270:dbl)
              n92 = local read "Frequency (Hz)"() -> (w266:dbl)
              n93 = local read "nu"() -> (w260:dbl)
              n94 = local read "Omega"() -> (w261:dbl)
              n95 = call-poly <vilib>:"Numeric Integration.vi"("integration method"=w272, "dt"=w270, "Input Array"=w273) -> ("result"=w269:dbl)  [unwired: 1 out]
              n96 = Subtract(x=w275, y=w276) -> (x-y=→"Phase Velocity _deg_":dbl)
              n97 = Square(x=w262) -> (x^2=w263:dbl)
              n98 = Divide(x=w269, y=2.0) -> (x/y=w267:dbl)
              "Stroke Length _m_" <- w267
              n99 = Multiply(x=w261, y=w263) -> (x*y=w259:dbl)
              n100 = Multiply(x=w266, y=w267) -> (x*y=w265:dbl)
              "Charicteristic Velocity m_s" <- w265
              n101 = Multiply(x=w265, y=w262) -> (x*y=w264:dbl)
              n102 = Divide(x=w264, y=w260) -> (x/y=w257:dbl)
              "Reynolds Number" <- w257
              n103 = Divide(x=w259, y=w260) -> (x/y=w258:dbl)
              n104 = Square Root(x=w258) -> (sqrt(x)=w255:dbl)
              "Stokes Number" <- w255
              n105 = Square(x=w255) -> (x^2=w256:dbl)
              n106 = Divide(x=w256, y=w257) -> (x/y=→"Strouhal Number":dbl)
              "Velocity m_s" <- w273
              "RMS Velocity m_s" <- w278
              "Max Velocity m_s" <- w277
            }
            frame "Mano (Pressure)" {
              n107 = Subtract(x=w281, y=w280) -> (x-y=→"Phase Pressure _deg_":dbl)
              "Pressure _Pa_" <- w284
              "RMS Pressure _Pa_" <- w283
              "Max Pressure _Pa_" <- w282
            }
            frame "No Match", Default {
              n108 = One Button Dialog(message="Error in Signal Analysis", button name ("OK")="STOP") -> (true=w286:bool)
              n109 = Stop(stop? (T)=w286) -> ()
            }
          }
        }
      }
      frame "LEM Calculations" {
        n110 = local read "Max Input Voltage _V_"() -> (w300:dbl)
        n111 = local read "Optimisation Type"() -> (w308:i32)
        n112 = local read "Strouhal Number"() -> (w313:dbl)
        n113 = local read "Max Velocity m_s"() -> (w290:dbl)
        n114 = Reciprocal(x=w313) -> (1/x=w312:dbl)
        "Formation Criteria" <- w312
        n115 = Divide(x=w300, y=20.0) -> (x/y=w289:dbl)
        n116 = Greater?(x=w312, y=0.16) -> (0:→"Jet Formation":bool)
        n117 = call "Read_Chan_Value_Gen.vi"("Desired Ch Names"=string[] ["Froude:NPL:Atmos_Press", "Aero_Tunnel:SmAD:Temp"], "Raw data file"=w316) -> ("Values"=w314:string[])  [unwired: 9 in]
        n118 = call "Get_Variable_Name.vi"("Data"=w289) -> ("Data Name(s)"=w305:string[])  [unwired: 24 in, 2 out]
        n119 = call "Get_Variable_Name.vi"("Data"=w290) -> ("Data Name(s)"=w306:string[])  [unwired: 24 in, 2 out]
        n120 = local read "Phase Pressure _deg_"() -> (w325:dbl)
        n121 = local read "Max Pressure _Pa_"() -> (w326:dbl)
        n122 = Fract/Exp String To Number(string=w314) -> (number=w334:dbl[])  [unwired: 3 in, 1 out]
        n123 = local read "Frequency (Hz)"() -> (w324:dbl)
        n124 = local read "Samps per cyle"() -> (w323:i32)
        n125 = Index Array(array=w334) -> (element #1=w331:dbl, element #2=w333:dbl)  [unwired: 2 in]
        n126 = Multiply(x=100.0 ("y"), y=w331) -> (x*y=w329:dbl)
        n127 = Add(x=w333, y=273.0) -> (x+y=w332:dbl)
        n128 = Bundle By Name(cluster=T8 {"R"=8.31451, "Mair"=0.0289645, "T"=293.0, "Patmos"=101325.0, "gamma"=1.4} ("Fluid Properties"), "Patmos"=w329, "T"=w332) -> (w327:T8)
        n129 = call "Get_LEM_Response.vi"("Frequency (Hz)"=w324, "Cavity Pressure Magnitude"=w326, "Cavity Pressure Phase"=w325, "Fluid Properties"=w327, "SJ Data IN"=w320) -> ("Phi"=w322:dbl, "Uo"=w307:dbl, "OmegaH"=w319:dbl)  [unwired: 2 in, 2 out]
        "LEM Phase Velocity _deg_" <- w322
        "LEM Max Velocity _ms_" <- w307
        n130 = case shown="1" w308 {
          tunnel: w307 -> [w342 _]
          tunnel: [w342 w343] -> w288
          frame 0, Default {
          }
          frame 1 {
            n131 = local read "Max Pressure _Pa_"() -> (w343:dbl)
          }
        }
        n132 = call "Get_Variable_Name.vi"("Data"=w288) -> ("Data Name(s)"=w304:string[])  [unwired: 24 in, 2 out]
        n133 = Build Array(w304, w305, w306) -> (w303:string[][])
        n134 = Replace Array Subset(array=w296, new element #1=w288, index (dim 0) #1=2 ("index (page)"), index (dim 1) #1=w292, index (dim 2) #1=w291, new element #2=w289, index (dim 0) #2=3 ("index (page)"), index (dim 1) #2=w292, index (dim 2) #2=w291) -> (w293:dbl[][][])
        "output array" <- w293
        "output array 2" <- w293
        n135 = for {
          tunnel: w303 -> [w341] mode=indexing
          tunnel: [w340] -> w302 mode=indexing
          tunnel: w297 -> [w339]
          n136 = Index Array(array=w341, index=w339) -> (element=w340:string)
        }
        "Output Data Names" <- w302
        n137 = call <vilib>:"Sine Pattern.vi"("phase(degrees)"=w322, "amplitude"=w307, "samples"=w323) -> ("Sinusoidal Pattern"=→"LEM Velocity _ms_":dbl[])  [unwired: 1 in, 1 out]
        n138 = Divide(x=w319, y=6.283185307179586) -> (x/y=→"Cavity:Helmholtz:Hz":dbl)
      }
      frame "Plot Graphs" {
        n139 = local read "Output Data Names"() -> (w355:string[])
        n140 = local read "Samps per cyle"() -> (w374:i32)
        n141 = call-poly <vilib>:"Ramp Pattern.vi"("exclude end?"=TRUE, "start"=0.0, "end"=360.0, "samples"=w374) -> ("Ramp Pattern"=w365:dbl[])  [unwired: 6 in, 1 out]
        "Phase Angle _deg_" <- w365
        n142 = Index Array(array=w355, index=w353) -> (element=w375:string)
        n143 = local read "LEM Velocity _ms_"() -> (w362:dbl[])
        n144 = local read "Input Voltage _V_"() -> (w370:dbl[])
        n145 = property on="Menu Ring" class="Ring (strict)"("Strings []"=w355) -> ()  [unwired: 2 in, 2 out]
        n146 = local read "Velocity m_s"() -> (w359:dbl[])
        n147 = local read "Pressure _Pa_"() -> (w368:dbl[])
        n148 = property on="Frequency Plot" class="XYGraph (strict)"("YScale.NameLbl.Text"=w375) -> ()  [unwired: 2 in, 2 out]
        n149 = call-poly <vilib>:"Quick Scale.vi"("X"=w362) -> ("Y[i]=X[i]/Max|X|"=w360:dbl[], "max|X|"=w361:dbl)  [unwired: 1 out]
        n150 = call-poly <vilib>:"Quick Scale.vi"("X"=w370) -> ("Y[i]=X[i]/Max|X|"=w369:dbl[])  [unwired: 2 out]
        n151 = call-poly <vilib>:"Quick Scale.vi"("X"=w368) -> ("Y[i]=X[i]/Max|X|"=w367:dbl[])  [unwired: 2 out]
        n152 = Divide(x=w359, y=w361) -> (x/y=w358:dbl[])
        n153 = local read "Sweep Frequency"() -> (w349:dbl[])
        n154 = Add(x=w353, y=u16 2) -> (x+y=w347:u16)
        n155 = Bundle("Ramp Pattern"=w365, "Y[i]=X[i]/Max|X|"=w369) -> (w376:T10)  [unwired: 1 in]
        n156 = Bundle("Ramp Pattern"=w365, "Y[i]=X[i]/Max|X|"=w367) -> (w379:T10)  [unwired: 1 in]
        n157 = Bundle("Ramp Pattern"=w365, w358) -> (w380:cluster{"Ramp Pattern":dbl[], dbl[]})  [unwired: 1 in]
        n158 = Bundle("Ramp Pattern"=w365, "Y[i]=X[i]/Max|X|"=w360) -> (w366:T10)  [unwired: 1 in]
        n159 = Index Array(array=w354, index (dim 0)=w347) -> (element=w345:dbl[][])  [unwired: 2 in]
        n160 = Build Array(w376, w379) -> (→"Pressure Plot":T11)
        n161 = Build Array(w376, w380, w366) -> (→"Velocity Plot":T11)
        n162 = for {
          tunnel: w349 -> [w384]
          tunnel: w345 -> [w383] mode=indexing
          tunnel: [w382] -> w344 mode=indexing
          n163 = Bundle("Sweep Frequency"=w384, w383) -> (w382:cluster{"Sweep Frequency":dbl[], dbl[]})  [unwired: 1 in]
        }
        "Frequency Plot" <- w344
        n164 = local read "Last Block in Genertation"() -> (w351:bool)
      }
      frame "PSO" {
        n165 = Equal To 0?(x=w389) -> (x = 0?=w388:bool)
        n166 = Index Array(array=w422) -> (element #1=w421:dbl[], element #2=w420:dbl[])  [unwired: 4 in]
        n167 = local read "Blocks per Generation"() -> (w395:i32)
        n168 = Index Array(array=w431) -> (element #1=w428:dbl[][], element #2=w427:dbl[][], element #3=w425:dbl[][], element #4=w423:dbl[][], element #5=w419:dbl[][])  [unwired: 15 in]
        "subarray" <- w427
        n169 = global read "DataTranslation_global.vi" "Amplitudes"() -> (w402:dbl[])
        n170 = Transpose 2D Array(2D array=w423) -> (transposed array=w387:dbl[][])
        n171 = Transpose 2D Array(2D array=w419) -> (transposed array=w418:dbl[][])
        n172 = Transpose 2D Array(2D array=w427) -> (transposed array=w426:dbl[][])
        n173 = Transpose 2D Array(2D array=w425) -> (transposed array=w424:dbl[][])
        n174 = Transpose 2D Array(2D array=w428) -> (transposed array=w385:dbl[][])
        n175 = case shown="False" w388 {
          tunnel: w387 -> [_ w439]
          tunnel: [w438 w439] -> w386
          tunnel: w385 -> [w438 _]
          frame False {
          }
          frame True {
          }
        }
        n176 = local read "Target Value"() -> (w429:dbl)
        n177 = for {
          tunnel: w429 -> [w458]
          tunnel: w386 -> [w457] mode=indexing
          tunnel: w426 -> [w456] mode=indexing
          tunnel: w424 -> [w455] mode=indexing
          tunnel: w387 -> [w448] mode=indexing
          tunnel: w421 -> [w454] mode=indexing
          tunnel: w420 -> [w453] mode=indexing
          tunnel: w418 -> [w449] mode=indexing
          tunnel: [w452] -> w417 mode=indexing
          tunnel: [w445] -> w416 mode=indexing
          tunnel: [w451] -> w414 mode=indexing
          tunnel: [w446] -> w413 mode=indexing
          tunnel: [w450] -> w412 mode=indexing
          tunnel: [w441] -> w407 mode=indexing
          tunnel: [w440] -> w408 mode=indexing
          n178 = call "Update_Best_Positions.vi"("Target Value"=w458, "Global Best Residual"=w454, "Global Best Position"=w453, "Particle Best Position"=w457, "Particle Best Residual"=w456, "Current Partical Value"=w455, "Current Particle Position"=w448) -> ("Updated Best Particle Residual"=w451:dbl[], "Updated Particle Best Position"=w446:dbl[], "Current Partical Value Out"=w450:dbl[], "Current Particle Position Out"=w447:dbl[], "Updated Global Best Residual"=w452:dbl, "Updated Global Best Position"=w445:dbl)  [unwired: 3 in]
          n179 = call "Calculate_New_Positions.vi"("C2"=0.1, "C1"=0.1, "Global best position"=w445, "Inertial Coefficient"=0.1, "Best Particle Position"=w446, "Current Particle Position"=w447, "Current Particle Velocity"=w449) -> ("Updated Particle Positions"=w441:dbl[], "Updated Particle Velocities"=w440:dbl[])  [unwired: 3 in]
        }
        n180 = Build Array(w417, w416) -> (w415:dbl[][])
        n181 = Increment(x=w389) -> (x+1=w391:i32)
        n182 = Multiply(x=w395, y=w391) -> (x*y=w394:i32)
        n183 = Increment(x=w394) -> (x+1=w400:i32)
        n184 = Transpose 2D Array(2D array=w414) -> (transposed array=w410:dbl[][])
        n185 = Transpose 2D Array(2D array=w413) -> (transposed array=w411:dbl[][])
        n186 = Transpose 2D Array(2D array=w412) -> (transposed array=w409:dbl[][])
        n187 = Transpose 2D Array(2D array=w407) -> (transposed array=w392:dbl[][])
        n188 = Transpose 2D Array(2D array=w408) -> (transposed array=w393:dbl[][])
        n189 = Array Size(array=w392) -> (size(s)=w404:i32[])
        n190 = Build Array(w411, w410, w409, w392, w393) -> (w430:dbl[][][])
        n191 = Index Array(array=w404) -> (element #1=w405:i32, element #2=w406:i32)  [unwired: 2 in]
        n192 = local read "Max Amp"() -> (w397:dbl)
        n193 = local read "Min Amp"() -> (w396:dbl)
        n194 = Multiply(x=w405, y=w406) -> (x*y=w403:i32)
        n195 = Reshape Array(w392, w403) -> (w398:dbl[])
        n196 = call <vilib>:"Y[i]=Clip{X[i]}.vi"("lower limit"=w396, "upper limit"=w397, "Input Array"=w398) -> ("Clipped Array"=w399:dbl[])  [unwired: 1 out]
        n197 = Replace Array Subset(array=w402, new element=w399, index=w400) -> (w390:dbl[])
        "Updated Amps" <- w390
        n198 = global write "DataTranslation_global.vi" "Amplitudes"(w390) -> ()
      }
      frame "End" {
      }
    }
  }
